vi "Launch Network.vi"(8 "error in (no error)":errorcluster, 11 "Cobra GUI in":refnum<class "Cobra GUI.lvclass">) -> (0 "error out":errorcluster, 3 "Cobra GUI out":refnum<class "Cobra GUI.lvclass">)   [LabVIEW 2019, in "Cobra GUI.lvlib" / "Cobra GUI.lvclass"]
uses:
  Cobra GUI.lvclass
  <vilib>/ActorFramework/Actor/Actor.lvclass
  Network Stream/Network Stream.lvclass
  GUI Messages/Receive NS connection Msg/Receive NS connection Msg.lvclass
  GUI Messages/Receive Dataset Msg/Receive Dataset Msg.lvclass
  C:/Working Copy/trunk/Modified Cobra Jung/Cobra/Cobra AF/Network Stream/Network Stream Messages/NS Connection Msg/NS Connection Msg.lvclass
  C:/Program Files (x86)/National Instruments/LabVIEW 2019/vi.lib/ActorFramework/Message/Message.lvclass
  C:/Working Copy/trunk/Modified Cobra Jung/Cobra/Cobra AF/Network Stream/Network Stream Messages/Dataset Msg/Dataset Msg.lvclass
  C:/Program Files (x86)/National Instruments/LabVIEW 2019/vi.lib/ActorFramework/Actor/Actor.lvclass
  C:/Program Files (x86)/National Instruments/LabVIEW 2019/vi.lib/MGI/Panel Manager/Panel Actor/Panel Actor/Panel Actor.lvclass
  C:/Program Files (x86)/National Instruments/LabVIEW 2019/vi.lib/MGI/Monitored Actor/Monitored Actor/Monitored Actor/Monitored Actor.lvclass
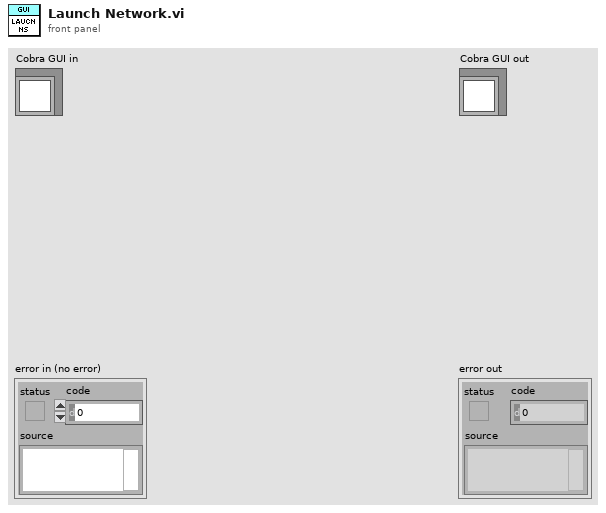
[diagram p1: front panel]
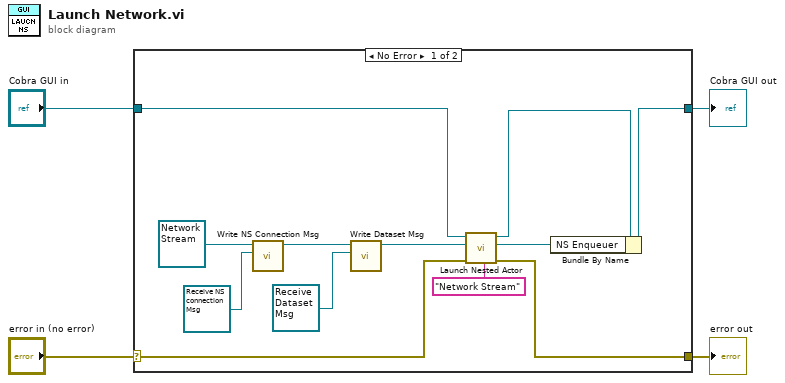
[diagram p0: block diagram]
diagram:
  n1 = case shown="No Error" "error in (no error)" {
    selector: "error in (no error)" -> [w13 w18]
    tunnel: [w11 w18] -> w3
    tunnel: [w5 w17] -> w1
    tunnel: "Cobra GUI in" -> [w12 w17]
    frame No Error {
      n2 = call "Write NS Connection Msg.vi"("GUI.lvlib:Network Stream.lvlib:NS Connection Msg.lvclass"=refnum<class "Receive NS connection Msg.lvclass"> refnum ("GUI.lvlib:Cobra GUI.lvlib:Receive NS connection Msg.lvclass"), "Network Stream in"=refnum<class "Network Stream.lvclass"> refnum ("GUI.lvlib:Network Stream.lvlib:Network Stream.lvclass")) -> ("Network Stream out"=w8:refnum<class "Network Stream.lvclass">)  [unwired: 9 in]
      n3 = call "Write Dataset Msg.vi"("GUI.lvlib:Network Stream.lvlib:Dataset Msg.lvclass"=refnum<class "Receive Dataset Msg.lvclass"> refnum ("GUI.lvlib:Cobra GUI.lvlib:Receive Dataset Msg.lvclass"), "Network Stream in"=w8) -> ("Network Stream out"=w7:refnum<class "Network Stream.lvclass">)  [unwired: 9 in]
      n4 = call <vilib>:"Launch Nested Actor.vi"("Debug Alias"="Network Stream", "error in (no error)"=w13, "Nested Actor"=w7, "Caller Actor in"=w12) -> ("error out"=w11:errorcluster, "Nested Actor's Enqueuer"=w6:refnum<class "Message Enqueuer.lvclass">, "Caller Actor out"=w10:refnum<class "Cobra GUI.lvclass">)  [unwired: 5 in]
      n5 = Bundle By Name(cluster=w10, "NS Enqueuer"=w6) -> (w5:refnum<class "Cobra GUI.lvclass">)
    }
    frame Error {
    }
  }
  "error out" <- w3
  "Cobra GUI out" <- w1
